vi "Set Started.vi"(8 "error in (no error)":errorcluster {"code" format="Error %.0f"}, 10 "Process":string, 11 "Progress Bar UI In":refnum<class "Progress Bar UI.lvclass">) -> (0 "error out":errorcluster {"code" format="Error %.0f"}, 3 "Progress Bar UI Out":refnum<class "Progress Bar UI.lvclass">)   [LabVIEW 2023, in "Progress Bar UI.lvclass"]
uses:
  Progress Bar UI.lvclass
  Progress Bar UI.lvclass/Progress Bar UI.ctl
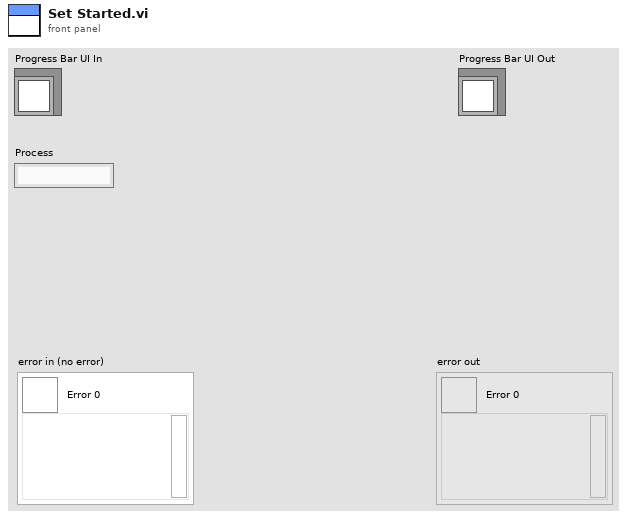
[diagram p1: front panel]
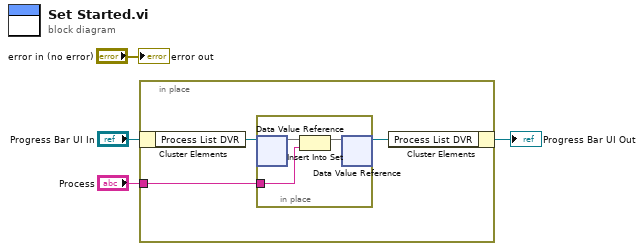
[diagram p0: block diagram]
diagram:
  n1 = in-place {
    in-place-border: "Process" -> [w7]
    n2 = in-place-cluster #1("Progress Bar UI In") -> ("Process List DVR"=w6:refnum<data-value>)
    n3 = in-place {
      in-place-border: w7 -> [w10]
      n4 = in-place-dvr #2(w6) -> (w9:set{string})  [unwired: 1 out]
      n5 = Insert Into Set(10:w10, 11:w9) -> (3:w8:set{string})  [unwired: 1 out]
      n6 = in-place-dvr #2(w8) -> (w5:refnum<data-value>)  [unwired: 1 out]
    }
    n7 = in-place-cluster #1("Process List DVR"=w5) -> (→"Progress Bar UI Out":refnum<class "Progress Bar UI.lvclass">)
  }
  "error out" <- "error in (no error)"
